vi "PR Run And Acquire Signal.vi"(2 "Number of Signals to be Acquired":i32, 3 "Length of Signal":i32) -> (0 "DataArray Out":i8[](array[numeric]), 1 "function return":bool)   [LabVIEW 2022 SP3, in "BS6006PRPLUS.lvlib"]
doc: "The function triggers the pulser/receiver starts to generate pulse and acquire the received signals. When the trigger source is internal, the number of pulses would be generated according to the setting of number of signals to be acquired.\n\n\n\nextern \"C\" BS6006PRPLUS_API bool __cdecl PR_RunAndAcquireSignal(char* DataArray);"
uses:
  BS6006PRPLUS.lvlib
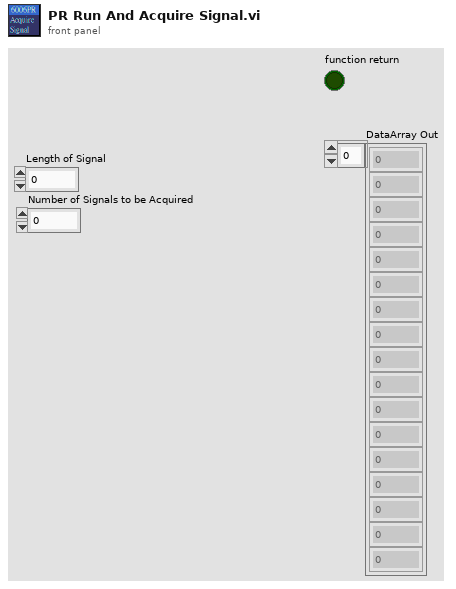
[diagram p1: front panel]
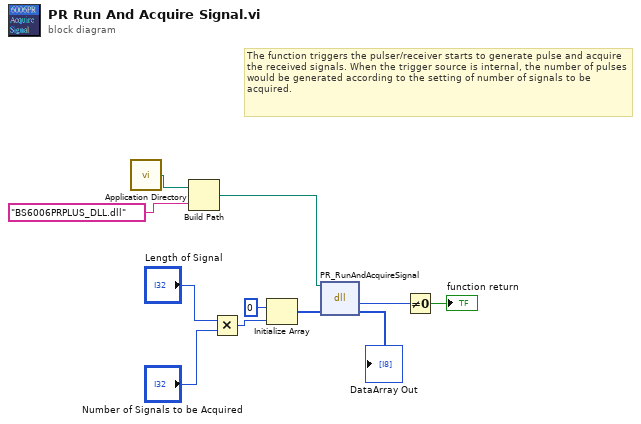
[diagram p0: block diagram]
diagram:
  # "The function triggers the pulser/receiver starts to generate pulse and acquire the received signals. When the trigger source is internal, the number of pulses would be generated according to the setting of number of signals to be acquired."
  n1 = call <vilib>:"Application Directory.vi"() -> ("Application Directory"=w3:path)
  n2 = Build Path(base path=w3, name or relative path="BS6006PRPLUS_DLL.dll") -> (appended path=w1:path)
  n3 = Multiply(x="Length of Signal", y="Number of Signals to be Acquired") -> (x*y=w8:i32)
  n4 = Initialize Array(i8 0 ("element"), w8) -> (w6:i8[])
  n5 = dll-call lib="E:/Broadsound_Program/PulserReceiver/6006PR PLUS/API/DLL/LabVIEW 15/VIs/BS6006PRPLUS_DLL.dll" fn="PR_RunAndAcquireSignal"(path in=w1, "DataArray"=w6) -> ("return type"=w10:u8, "DataArray"=→"DataArray Out":i8[])  [unwired: 2 in, 2 out]
  n6 = Not Equal To 0?(x=w10) -> (x != 0?=→"function return":bool)
